vi "E3_2.vi"   [LabVIEW 2017]
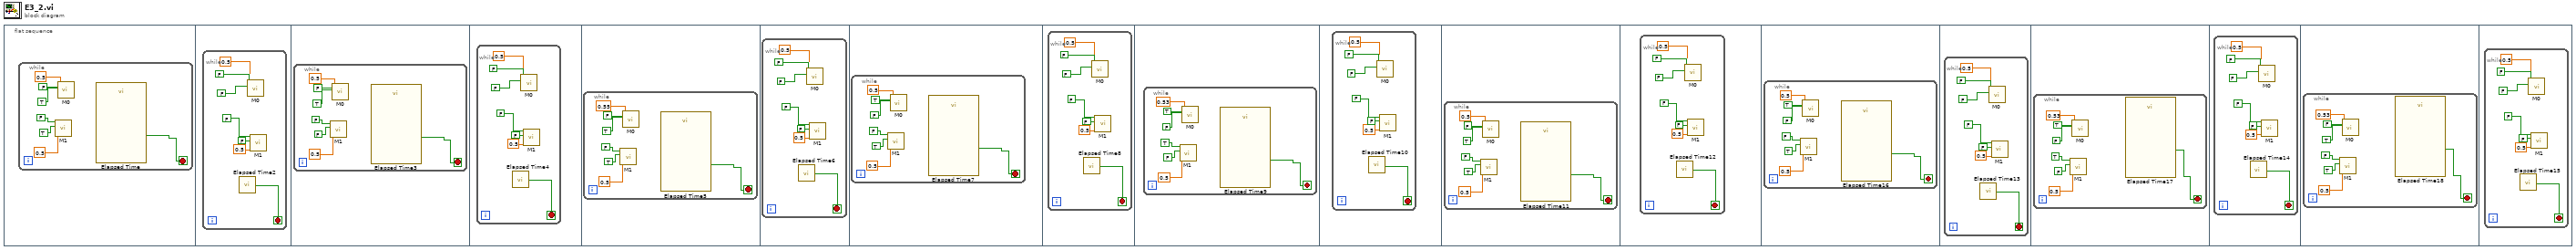
[diagram p0: block diagram]
diagram:
  n1 = flat-sequence {
    frame #0 {
      n2 = while {
        stop <- w1 stop-if-true
        n3 = call "M1.vi"("Duty Cycle"=0.5, "вперед"=TRUE, "назад"=FALSE) -> ()  [unwired: 8 in, 1 out]
        n4 = call "M0.vi"("Duty Cycle"=0.5, "вперед"=TRUE, "назад"=FALSE) -> ()  [unwired: 8 in, 1 out]
        n5 = call "Elapsed Time"() -> ("Time has Elapsed"=w1:bool)  [unwired: 12 in, 7 out]
      }
    }
    frame #1 {
      n6 = while {
        stop <- w8 stop-if-true
        n7 = call "Elapsed Time2"() -> ("Time has Elapsed"=w8:bool)  [unwired: 12 in, 7 out]
        n8 = call "M0.vi"("Duty Cycle"=0.5, "вперед"=FALSE, "назад"=FALSE) -> ()  [unwired: 8 in, 1 out]
        n9 = call "M1.vi"("Duty Cycle"=0.5, "вперед"=FALSE, "назад"=FALSE) -> ()  [unwired: 8 in, 1 out]
      }
    }
    frame #2 {
      n10 = while {
        stop <- w15 stop-if-true
        n11 = call "M1.vi"("Duty Cycle"=0.5, "вперед"=FALSE, "назад"=FALSE) -> ()  [unwired: 8 in, 1 out]
        n12 = call "M0.vi"("Duty Cycle"=0.5, "вперед"=TRUE, "назад"=FALSE) -> ()  [unwired: 8 in, 1 out]
        n13 = call "Elapsed Time3"() -> ("Time has Elapsed"=w15:bool)  [unwired: 12 in, 7 out]
      }
    }
    frame #3 {
      n14 = while {
        stop <- w22 stop-if-true
        n15 = call "Elapsed Time4"() -> ("Time has Elapsed"=w22:bool)  [unwired: 12 in, 7 out]
        n16 = call "M0.vi"("Duty Cycle"=0.5, "вперед"=FALSE, "назад"=FALSE) -> ()  [unwired: 8 in, 1 out]
        n17 = call "M1.vi"("Duty Cycle"=0.5, "вперед"=FALSE, "назад"=FALSE) -> ()  [unwired: 8 in, 1 out]
      }
    }
    frame #4 {
      n18 = while {
        stop <- w29 stop-if-true
        n19 = call "M1.vi"("Duty Cycle"=0.5, "вперед"=TRUE, "назад"=FALSE) -> ()  [unwired: 8 in, 1 out]
        n20 = call "M0.vi"("Duty Cycle"=0.55, "вперед"=TRUE, "назад"=FALSE) -> ()  [unwired: 8 in, 1 out]
        n21 = call "Elapsed Time5"() -> ("Time has Elapsed"=w29:bool)  [unwired: 12 in, 7 out]
      }
    }
    frame #5 {
      n22 = while {
        stop <- w36 stop-if-true
        n23 = call "Elapsed Time6"() -> ("Time has Elapsed"=w36:bool)  [unwired: 12 in, 7 out]
        n24 = call "M0.vi"("Duty Cycle"=0.5, "вперед"=FALSE, "назад"=FALSE) -> ()  [unwired: 8 in, 1 out]
        n25 = call "M1.vi"("Duty Cycle"=0.5, "вперед"=FALSE, "назад"=FALSE) -> ()  [unwired: 8 in, 1 out]
      }
    }
    frame #6 {
      n26 = while {
        stop <- w43 stop-if-true
        n27 = call "M1.vi"("Duty Cycle"=0.5, "вперед"=TRUE, "назад"=FALSE) -> ()  [unwired: 8 in, 1 out]
        n28 = call "M0.vi"("Duty Cycle"=0.5, "вперед"=FALSE, "назад"=TRUE) -> ()  [unwired: 8 in, 1 out]
        n29 = call "Elapsed Time7"() -> ("Time has Elapsed"=w43:bool)  [unwired: 12 in, 7 out]
      }
    }
    frame #7 {
      n30 = while {
        stop <- w50 stop-if-true
        n31 = call "Elapsed Time8"() -> ("Time has Elapsed"=w50:bool)  [unwired: 12 in, 7 out]
        n32 = call "M0.vi"("Duty Cycle"=0.5, "вперед"=FALSE, "назад"=FALSE) -> ()  [unwired: 8 in, 1 out]
        n33 = call "M1.vi"("Duty Cycle"=0.5, "вперед"=FALSE, "назад"=FALSE) -> ()  [unwired: 8 in, 1 out]
      }
    }
    frame #8 {
      n34 = while {
        stop <- w57 stop-if-true
        n35 = call "M1.vi"("Duty Cycle"=0.5, "вперед"=FALSE, "назад"=TRUE) -> ()  [unwired: 8 in, 1 out]
        n36 = call "M0.vi"("Duty Cycle"=0.53, "вперед"=FALSE, "назад"=TRUE) -> ()  [unwired: 8 in, 1 out]
        n37 = call "Elapsed Time9"() -> ("Time has Elapsed"=w57:bool)  [unwired: 12 in, 7 out]
      }
    }
    frame #9 {
      n38 = while {
        stop <- w64 stop-if-true
        n39 = call "Elapsed Time10"() -> ("Time has Elapsed"=w64:bool)  [unwired: 12 in, 7 out]
        n40 = call "M0.vi"("Duty Cycle"=0.5, "вперед"=FALSE, "назад"=FALSE) -> ()  [unwired: 8 in, 1 out]
        n41 = call "M1.vi"("Duty Cycle"=0.5, "вперед"=FALSE, "назад"=FALSE) -> ()  [unwired: 8 in, 1 out]
      }
    }
    frame #10 {
      n42 = while {
        stop <- w71 stop-if-true
        n43 = call "M1.vi"("Duty Cycle"=0.5, "вперед"=TRUE, "назад"=FALSE) -> ()  [unwired: 8 in, 1 out]
        n44 = call "M0.vi"("Duty Cycle"=0.5, "вперед"=TRUE, "назад"=FALSE) -> ()  [unwired: 8 in, 1 out]
        n45 = call "Elapsed Time11"() -> ("Time has Elapsed"=w71:bool)  [unwired: 12 in, 7 out]
      }
    }
    frame #11 {
      n46 = while {
        stop <- w78 stop-if-true
        n47 = call "Elapsed Time12"() -> ("Time has Elapsed"=w78:bool)  [unwired: 12 in, 7 out]
        n48 = call "M0.vi"("Duty Cycle"=0.5, "вперед"=FALSE, "назад"=FALSE) -> ()  [unwired: 8 in, 1 out]
        n49 = call "M1.vi"("Duty Cycle"=0.5, "вперед"=FALSE, "назад"=FALSE) -> ()  [unwired: 8 in, 1 out]
      }
    }
    frame #12 {
      n50 = while {
        stop <- w85 stop-if-true
        n51 = call "M1.vi"("Duty Cycle"=0.5, "вперед"=TRUE, "назад"=FALSE) -> ()  [unwired: 8 in, 1 out]
        n52 = call "M0.vi"("Duty Cycle"=0.5, "вперед"=FALSE, "назад"=TRUE) -> ()  [unwired: 8 in, 1 out]
        n53 = call "Elapsed Time16"() -> ("Time has Elapsed"=w85:bool)  [unwired: 12 in, 7 out]
      }
    }
    frame #13 {
      n54 = while {
        stop <- w92 stop-if-true
        n55 = call "Elapsed Time13"() -> ("Time has Elapsed"=w92:bool)  [unwired: 12 in, 7 out]
        n56 = call "M0.vi"("Duty Cycle"=0.5, "вперед"=FALSE, "назад"=FALSE) -> ()  [unwired: 8 in, 1 out]
        n57 = call "M1.vi"("Duty Cycle"=0.5, "вперед"=FALSE, "назад"=FALSE) -> ()  [unwired: 8 in, 1 out]
      }
    }
    frame #14 {
      n58 = while {
        stop <- w99 stop-if-true
        n59 = call "M1.vi"("Duty Cycle"=0.5, "вперед"=FALSE, "назад"=TRUE) -> ()  [unwired: 8 in, 1 out]
        n60 = call "M0.vi"("Duty Cycle"=0.53, "вперед"=FALSE, "назад"=TRUE) -> ()  [unwired: 8 in, 1 out]
        n61 = call "Elapsed Time17"() -> ("Time has Elapsed"=w99:bool)  [unwired: 12 in, 7 out]
      }
    }
    frame #15 {
      n62 = while {
        stop <- w106 stop-if-true
        n63 = call "Elapsed Time14"() -> ("Time has Elapsed"=w106:bool)  [unwired: 12 in, 7 out]
        n64 = call "M0.vi"("Duty Cycle"=0.5, "вперед"=FALSE, "назад"=FALSE) -> ()  [unwired: 8 in, 1 out]
        n65 = call "M1.vi"("Duty Cycle"=0.5, "вперед"=FALSE, "назад"=FALSE) -> ()  [unwired: 8 in, 1 out]
      }
    }
    frame #16 {
      n66 = while {
        stop <- w113 stop-if-true
        n67 = call "M1.vi"("Duty Cycle"=0.5, "вперед"=TRUE, "назад"=FALSE) -> ()  [unwired: 8 in, 1 out]
        n68 = call "M0.vi"("Duty Cycle"=0.53, "вперед"=TRUE, "назад"=FALSE) -> ()  [unwired: 8 in, 1 out]
        n69 = call "Elapsed Time18"() -> ("Time has Elapsed"=w113:bool)  [unwired: 12 in, 7 out]
      }
    }
    frame #17 {
      n70 = while {
        stop <- w120 stop-if-true
        n71 = call "Elapsed Time15"() -> ("Time has Elapsed"=w120:bool)  [unwired: 12 in, 7 out]
        n72 = call "M0.vi"("Duty Cycle"=0.5, "вперед"=FALSE, "назад"=FALSE) -> ()  [unwired: 8 in, 1 out]
        n73 = call "M1.vi"("Duty Cycle"=0.5, "вперед"=FALSE, "назад"=FALSE) -> ()  [unwired: 8 in, 1 out]
      }
    }
  }
